vi "Send SetAOTask.vi"(6 "AOChConfigs":refnum<class "AOChConfig.lvclass">[](array[class]), 7 "Priority":T1=enum."Normal" caption="Message Priority (Normal)", 8 "error in (no error)":errorcluster, 9 "AO Waveforms":waveform(dbl)[](array[waveform]), 10 "AO DAQChannels":tag[](array[tag]), 11 "Message Enqueuer in":refnum<class "Message Enqueuer.lvclass">) -> (0 "error out":errorcluster, 3 "Message Enqueuer out":refnum<class "Message Enqueuer.lvclass">)   [LabVIEW 2015, in "IO Device.lvlib" / "SetAOTask Msg.lvclass"]
doc: "Sends the <b>SetAOTask Msg.lvclass</b> message.\n\nThis message will call <b>SetAOTask.vi</b> on the <b>IO Device.lvlib:IO Device.lvclass</b> actor.\n\n<b>SetAOTask.vi Description</b>"
uses:
  SetAOTask Msg.lvclass
  <vilib>/ActorFramework/Message Enqueuer/Message Enqueuer.lvclass
  <vilib>/ActorFramework/Message Enqueuer/Message Priority.ctl
  Analog Output Channel/AOChConfig.lvclass
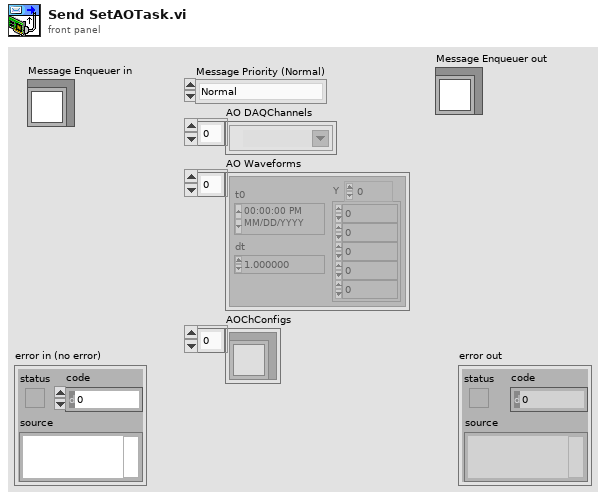
[diagram p1: front panel]
types:
  T1 = typedef "Actor Framework.lvlib/Message Enqueuer.lvclass/Message Priority.ctl" = enum16{"Low", "Normal", "High"}
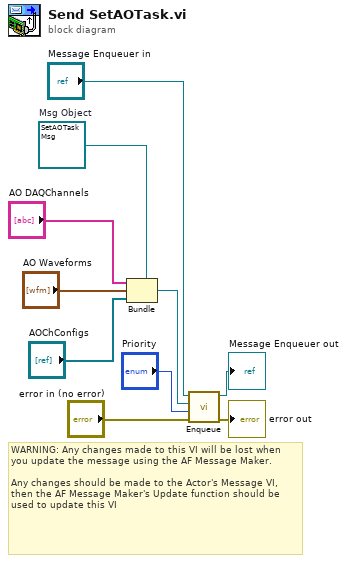
[diagram p0: block diagram]
diagram:
  w7 = refnum<class "SetAOTask Msg.lvclass"> refnum  # Msg Object
  # "WARNING: Any changes made to this VI will be lost when you update the message using the AF Message Maker.\n\nAny changes should be made to the Actor's Message VI, then the AF Message Maker's Update function should be used to update this VI"
  n1 = Bundle(cluster=w7, "AO DAQChannels", "AO Waveforms", "AOChConfigs") -> (w2:refnum<class "SetAOTask Msg.lvclass">)
  n2 = call <vilib>:"Enqueue.vi"("error in (no error)"="error in (no error)", "Message Priority (Normal)"="Priority", "Message"=w2, "Message Enqueuer in"="Message Enqueuer in") -> ("error out"=→"error out":errorcluster, "Message Enqueuer out"=→"Message Enqueuer out":refnum<class "Message Enqueuer.lvclass">)  [unwired: 6 in]
